vi "Read_currentNumber.vi"(8 "error in (no error)":errorcluster, 11 "FactoryTcpServer in":refnum<class "FactoryTcpServer.lvclass">) -> (0 "error out":errorcluster, 2 "currentNumber":i32, 3 "FactoryTcpServer out":refnum<class "FactoryTcpServer.lvclass">)   [LabVIEW 2018, in "FactoryTcpServer.lvclass"]
doc: "Read the currentNumber."
uses:
  FactoryTcpServer.lvclass
  FactoryTcpServer.lvclass/FactoryTcpServer.ctl
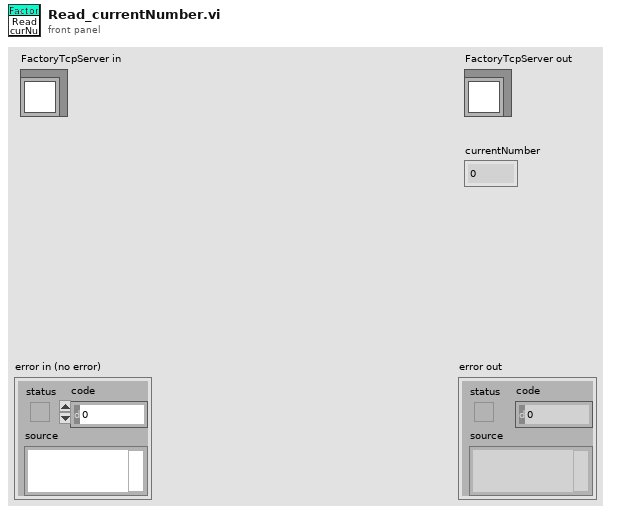
[diagram p1: front panel]
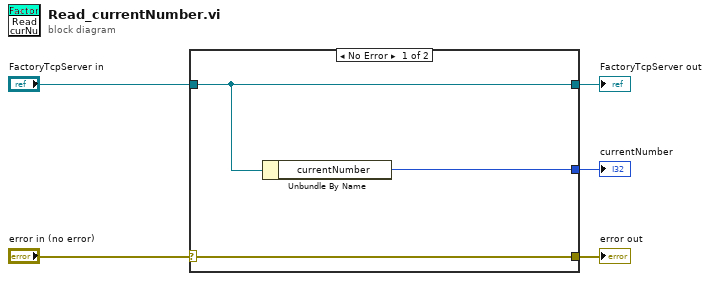
[diagram p0: block diagram]
diagram:
  n1 = case shown="No Error" "error in (no error)" {
    selector: "error in (no error)" -> [w8 w9]
    tunnel: [w8 w9] -> w4
    tunnel: [w7 w10] -> w2
    tunnel: "FactoryTcpServer in" -> [w7 w10]
    tunnel: [w6 _] -> w1
    frame No Error {
      n2 = Unbundle By Name(w7) -> ("currentNumber"=w6:i32)
    }
    frame Error {
    }
  }
  "error out" <- w4
  "FactoryTcpServer out" <- w2
  "currentNumber" <- w1
